vi "TRITON_REMOTE_INTERFACE_EXAMPLE.vi"() -> ()   [LabVIEW 2018]
panel:
  out "Connection Open":bool
  out "Trimmed String":string
  in  "Stop Communication":bool
  out "Response String":string
  in  "Send Command":bool
  in  "Command to send":string
  out "error out":errorcluster
  in  "Mode":T1(ring)=enum."Immediate"
  in  "Bytes to Read":i32=5000
  in  "IP Address":string="192.168.0.2"
  in  "Remote Port":i32=33576
  in  "Timeout":i32=10000
  in  "Open Connection":bool
  in  "error in (no error)":errorcluster
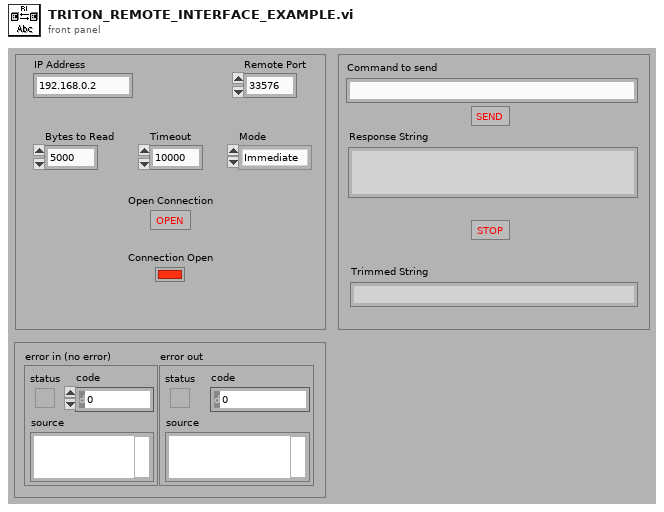
[diagram p1: front panel]
types:
  T1 = enum16{"Standard", "Buffered", "CRLF", "Immediate"}
  T2 = cluster{"Mode":enum16{"Standard", "Buffered", "CRLF", "Immediate"}, "Bytes to Read":i32, "IP Address":string, "Remote Port":i32, "Timeout":i32}
  T3 = cluster{"Mode":enum16{"Standard", "Buffered", "CRLF", "Immediate"}, "Bytes to Read":i32, "IP Address":string, "Remote Port":i32, "Timeout":i32, "connection ID":refnum<k5>}
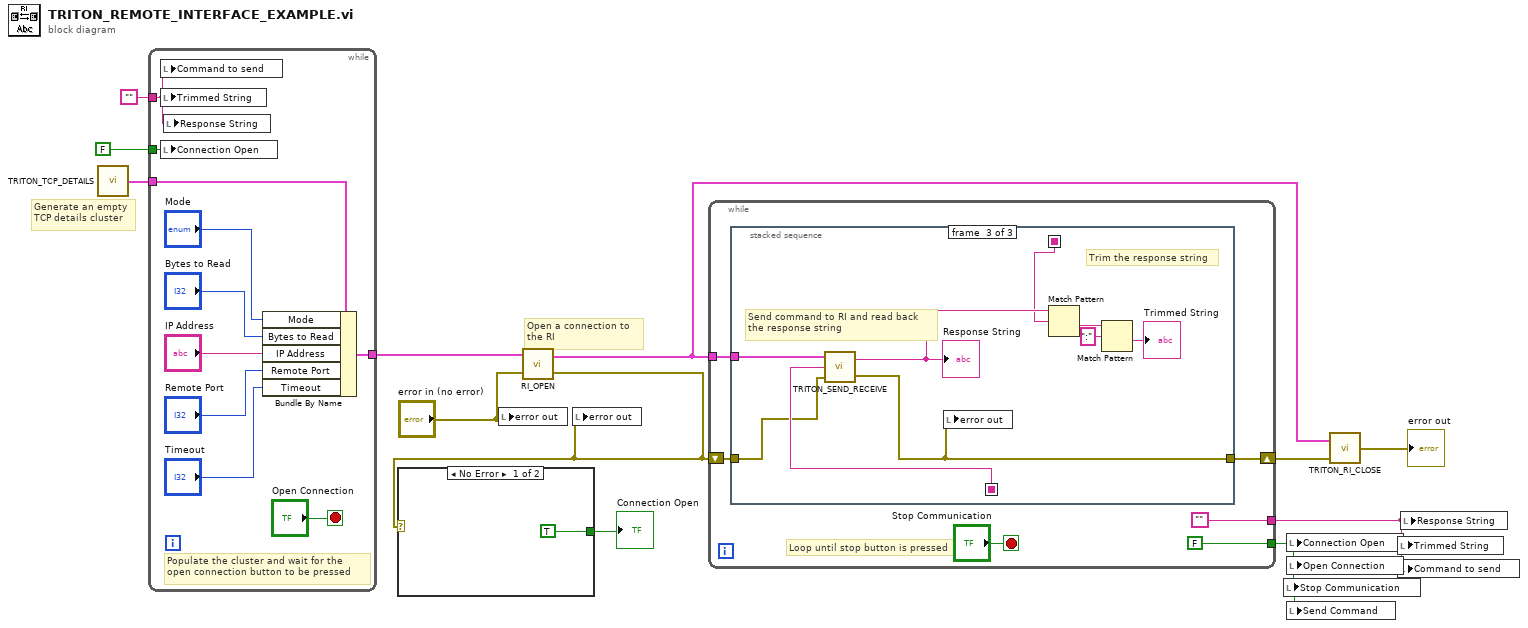
[diagram p0: block diagram]
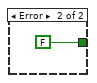
[diagram p2: hidden frame]
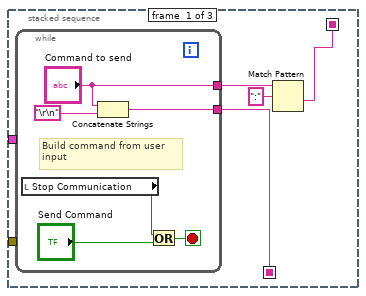
[diagram p3: hidden frame]
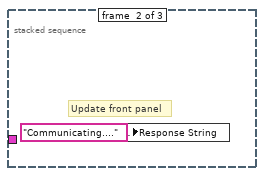
[diagram p4: hidden frame]
diagram:
  # "Open a connection to\nthe RI"
  # "Generate an empty\nTCP details cluster"
  n1 = call "TRITON_TCP_DETAILS.vi"() -> ("Cluster"=w12:T2)
  n2 = while {
    tunnel: w12 -> [w22]
    tunnel: [w15] -> w5
    tunnel: FALSE -> [w14]
    tunnel: "" -> [w13]
    stop <- "Open Connection" stop-if-true
    # "Populate the cluster and wait for the\nopen connection button to be pressed"
    n3 = local write "Command to send"(w13) -> ()
    n4 = local write "Trimmed String"(w13) -> ()
    n5 = local write "Connection Open"(w14) -> ()
    n6 = local write "Response String"(w13) -> ()
    n7 = Bundle By Name(cluster=w22, "Mode"="Mode", "Bytes to Read"="Bytes to Read", "IP Address"="IP Address", "Remote Port"="Remote Port", "Timeout"="Timeout") -> (w15:T2)
  }
  n8 = local write "error out"("error in (no error)") -> ()
  n9 = call "RI_OPEN.vi"("error in (no error)"="error in (no error)", "Cluster"=w5) -> ("error out"=w4:errorcluster, "output cluster"=w1:T3)
  n10 = case shown="No Error" w4 {
    tunnel: [TRUE FALSE] -> w10
    frame No Error {
    }
    frame Error {
    }
  }
  "Connection Open" <- w10
  n11 = local write "error out"(w4) -> ()
  n12 = while {
    shift-right: [w28] -> w3
    shift-left: w4 -> [w29]
    tunnel: [""] -> w6
    tunnel: [FALSE] -> w8
    tunnel: w1 -> [w25]
    stop <- "Stop Communication" stop-if-true
    # "Loop until stop button is pressed"
    n13 = stacked-sequence {
      seq-local: [w34 _ _] -> [_ _ w50]
      seq-local: [w31 _ _] -> [_ _ w46]
      tunnel: w29 -> [_ _ w49]
      tunnel: [_ _ w48] -> w28
      tunnel: w25 -> [_ _ w42]
      frame #0 {
        n14 = while {
          tunnel: [w36] -> w34
          tunnel: ["Command to send"] -> w33
          stop <- w38 stop-if-true
          # "Build command from user\ninput"
          n15 = local read "Stop Communication"() -> (w37:bool)
          n16 = Concatenate Strings("Command to send", "\r\n") -> (w36:string)
          n17 = Or(x=w37, y="Send Command") -> (x .or. y?=w38:bool)
        }
        n18 = Match Pattern(string=w33, regular expression=":") -> (after substring=w31:string)  [unwired: 1 in, 3 out]
      }
      frame #1 {
        # "Update front panel"
        n19 = local write "Response String"("Communicating...." ("Response String")) -> ()
      }
      frame #2 {
        # "Trim the response string"
        # "Send command to RI and read back\nthe response string"
        n20 = call "TRITON_SEND_RECEIVE.vi"("error in (no error)"=w49, "Command String"=w50, "Communication Cluster"=w42) -> ("error out"=w48:errorcluster, "Response String"=w47:string)
        "Response String" <- w47
        n21 = local write "error out"(w48) -> ()
        n22 = Match Pattern(string=w47, regular expression=w46) -> (after substring=w45:string)  [unwired: 1 in, 3 out]
        n23 = Match Pattern(string=w45, regular expression=":") -> (after substring=→"Trimmed String":string)  [unwired: 1 in, 3 out]
      }
    }
  }
  n24 = local write "Stop Communication"(w8) -> ()
  n25 = local write "Connection Open"(w8) -> ()
  n26 = local write "Open Connection"(w8) -> ()
  n27 = local write "Send Command"(w8) -> ()
  n28 = call "TRITON_RI_CLOSE.vi"("error in (no error)"=w3, "Communication Cluster"=w1) -> ("error out"=→"error out":errorcluster)
  n29 = local write "Trimmed String"(w6) -> ()
  n30 = local write "Command to send"(w6) -> ()
  n31 = local write "Response String"(w6) -> ()
